vi "MH_AllDllFunctions_AnyThread.vi"   [LabVIEW 2020]
uses:
  mhlib_x86_x64_AnyThread.llb/MH_DllPath_global.vi
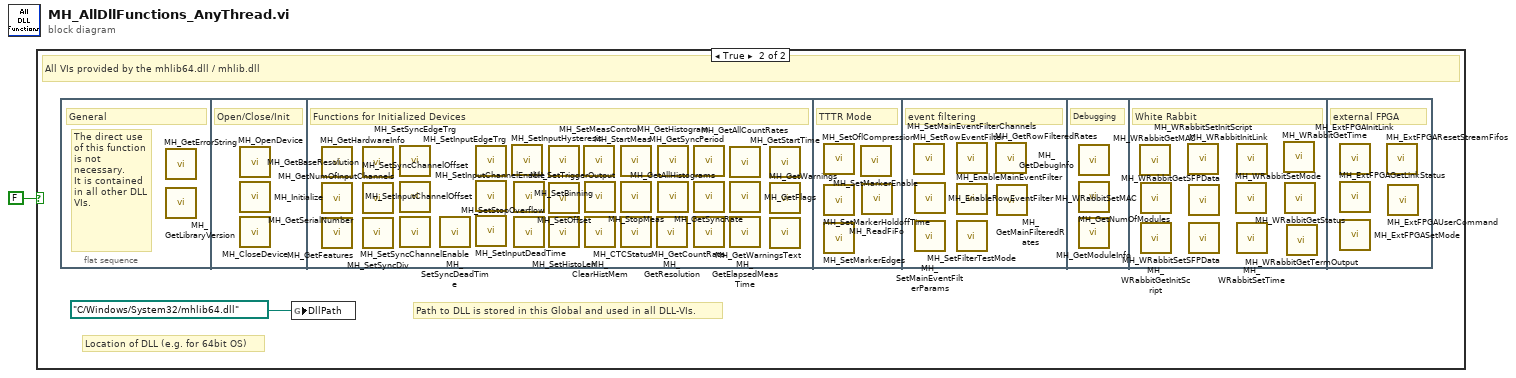
[diagram p0: block diagram]
diagram:
  n1 = case shown="True" FALSE {
    frame False {
    }
    frame True {
      # "Location of DLL (e.g. for 64bit OS)"
      # "Path to DLL is stored in this Global and used in all DLL-VIs."
      # "All VIs provided by the mhlib64.dll / mhlib.dll"
      n2 = flat-sequence {
        frame #0 {
          # "The direct use of this function is not necessary.\nIt is contained in all other DLL VIs."
          # "General"
          n3 = call "MH_GetErrorString.vi"() -> ()  [unwired: 9 in, 3 out]
          n4 = call "MH_GetLibraryVersion.vi"() -> ()  [unwired: 9 in, 3 out]
        }
        frame #1 {
          # "Open/Close/Init"
          n5 = call "MH_OpenDevice.vi"() -> ()  [unwired: 9 in, 3 out]
          n6 = call "MH_Initialize.vi"() -> ()  [unwired: 10 in, 2 out]
          n7 = call "MH_CloseDevice.vi"() -> ()  [unwired: 10 in, 2 out]
        }
        frame #2 {
          # "Functions for Initialized Devices"
          n8 = call "MH_GetHardwareInfo.vi"() -> ()  [unwired: 7 in, 5 out]
          n9 = call "MH_GetSerialNumber.vi"() -> ()  [unwired: 9 in, 3 out]
          n10 = call "MH_GetFeatures.vi"() -> ()  [unwired: 9 in, 3 out]
          n11 = call "MH_GetBaseResolution.vi"() -> ()  [unwired: 8 in, 4 out]
          n12 = call "MH_GetNumOfInputChannels.vi"() -> ()  [unwired: 9 in, 3 out]
          n13 = call "MH_SetSyncDiv.vi"() -> ()  [unwired: 10 in, 2 out]
          n14 = call "MH_SetSyncEdgeTrg.vi"() -> ()  [unwired: 10 in, 2 out]
          n15 = call "MH_SetSyncChannelOffset.vi"() -> ()  [unwired: 10 in, 2 out]
          n16 = call "MH_SetSyncChannelEnable.vi"() -> ()  [unwired: 10 in, 2 out]
          n17 = call "MH_SetSyncDeadTime.vi"() -> ()  [unwired: 10 in, 2 out]
          n18 = call "MH_SetInputEdgeTrg.vi"() -> ()  [unwired: 10 in, 2 out]
          n19 = call "MH_SetInputChannelOffset.vi"() -> ()  [unwired: 10 in, 2 out]
          n20 = call "MH_SetInputDeadTime.vi"() -> ()  [unwired: 10 in, 2 out]
          n21 = call "MH_SetInputHysteresis.vi"() -> ()  [unwired: 10 in, 2 out]
          n22 = call "MH_SetInputChannelEnable.vi"() -> ()  [unwired: 10 in, 2 out]
          n23 = call "MH_SetStopOverflow.vi"() -> ()  [unwired: 10 in, 2 out]
          n24 = call "MH_SetBinning.vi"() -> ()  [unwired: 10 in, 2 out]
          n25 = call "MH_SetOffset.vi"() -> ()  [unwired: 10 in, 2 out]
          n26 = call "MH_SetHistoLen.vi"() -> ()  [unwired: 9 in, 3 out]
          n27 = call "MH_SetMeasControl.vi"() -> ()  [unwired: 10 in, 2 out]
          n28 = call "MH_SetTriggerOutput.vi"() -> ()  [unwired: 10 in, 2 out]
          n29 = call "MH_ClearHistMem.vi"() -> ()  [unwired: 10 in, 2 out]
          n30 = call "MH_StartMeas.vi"() -> ()  [unwired: 10 in, 2 out]
          n31 = call "MH_StopMeas.vi"() -> ()  [unwired: 10 in, 2 out]
          n32 = call "MH_CTCStatus.vi"() -> ()  [unwired: 9 in, 3 out]
          n33 = call "MH_GetResolution.vi"() -> ()  [unwired: 9 in, 3 out]
          n34 = call "MH_GetHistogram.vi"() -> ()  [unwired: 9 in, 3 out]
          n35 = call "MH_GetAllHistograms.vi"() -> ()  [unwired: 9 in, 3 out]
          n36 = call "MH_GetSyncPeriod.vi"() -> ()  [unwired: 9 in, 3 out]
          n37 = call "MH_GetSyncRate.vi"() -> ()  [unwired: 9 in, 3 out]
          n38 = call "MH_GetCountRate.vi"() -> ()  [unwired: 9 in, 3 out]
          n39 = call "MH_GetAllCountRates.vi"() -> ()  [unwired: 8 in, 4 out]
          n40 = call "MH_GetFlags.vi"() -> ()  [unwired: 9 in, 3 out]
          n41 = call "MH_GetElapsedMeasTime.vi"() -> ()  [unwired: 9 in, 3 out]
          n42 = call "MH_GetStartTime.vi"() -> ()  [unwired: 7 in, 5 out]
          n43 = call "MH_GetWarnings.vi"() -> ()  [unwired: 9 in, 3 out]
          n44 = call "MH_GetWarningsText.vi"() -> ()  [unwired: 9 in, 3 out]
        }
        frame #3 {
          # "TTTR Mode"
          n45 = call "MH_SetOflCompression.vi"() -> ()  [unwired: 10 in, 2 out]
          n46 = call "MH_SetMarkerHoldoffTime.vi"() -> ()  [unwired: 10 in, 2 out]
          n47 = call "MH_SetMarkerEdges.vi"() -> ()  [unwired: 10 in, 2 out]
          n48 = call "MH_SetMarkerEnable.vi"() -> ()  [unwired: 10 in, 2 out]
          n49 = call "MH_ReadFiFo.vi"() -> ()  [unwired: 8 in, 4 out]
        }
        frame #4 {
          # "event filtering"
          n50 = call "MH_SetRowEventFilter.vi"() -> ()  [unwired: 10 in, 2 out]
          n51 = call "MH_EnableRowEventFilter.vi"() -> ()  [unwired: 10 in, 2 out]
          n52 = call "MH_SetMainEventFilterParams.vi"() -> ()  [unwired: 10 in, 2 out]
          n53 = call "MH_SetMainEventFilterChannels.vi"() -> ()  [unwired: 10 in, 2 out]
          n54 = call "MH_EnableMainEventFilter.vi"() -> ()  [unwired: 10 in, 2 out]
          n55 = call "MH_SetFilterTestMode.vi"() -> ()  [unwired: 10 in, 2 out]
          n56 = call "MH_GetRowFilteredRates.vi"() -> ()  [unwired: 8 in, 4 out]
          n57 = call "MH_GetMainFilteredRates.vi"() -> ()  [unwired: 8 in, 4 out]
        }
        frame #5 {
          # "Debugging"
          n58 = call "MH_GetDebugInfo.vi"() -> ()  [unwired: 9 in, 3 out]
          n59 = call "MH_GetNumOfModules.vi"() -> ()  [unwired: 9 in, 3 out]
          n60 = call "MH_GetModuleInfo.vi"() -> ()  [unwired: 8 in, 4 out]
        }
        frame #6 {
          # "White Rabbit"
          n61 = call "MH_WRabbitGetMAC.vi"() -> ()  [unwired: 9 in, 3 out]
          n62 = call "MH_WRabbitSetMAC.vi"() -> ()  [unwired: 10 in, 2 out]
          n63 = call "MH_WRabbitGetInitScript.vi"() -> ()  [unwired: 9 in, 3 out]
          n64 = call "MH_WRabbitSetInitScript.vi"() -> ()  [unwired: 10 in, 2 out]
          n65 = call "MH_WRabbitGetSFPData.vi"() -> ()  [unwired: 6 in, 6 out]
          n66 = call "MH_WRabbitSetSFPData.vi"() -> ()  [unwired: 10 in, 2 out]
          n67 = call "MH_WRabbitSetMode.vi"() -> ()  [unwired: 10 in, 2 out]
          n68 = call "MH_WRabbitInitLink.vi"() -> ()  [unwired: 10 in, 2 out]
          n69 = call "MH_WRabbitSetTime.vi"() -> ()  [unwired: 10 in, 2 out]
          n70 = call "MH_WRabbitGetTime.vi"() -> ()  [unwired: 8 in, 4 out]
          n71 = call "MH_WRabbitGetStatus.vi"() -> ()  [unwired: 9 in, 3 out]
          n72 = call "MH_WRabbitGetTermOutput.vi"() -> ()  [unwired: 8 in, 4 out]
        }
        frame #7 {
          # "external FPGA"
          n73 = call "MH_ExtFPGAInitLink.vi"() -> ()  [unwired: 10 in, 2 out]
          n74 = call "MH_ExtFPGAGetLinkStatus.vi"() -> ()  [unwired: 9 in, 3 out]
          n75 = call "MH_ExtFPGASetMode.vi"() -> ()  [unwired: 10 in, 2 out]
          n76 = call "MH_ExtFPGAResetStreamFifos.vi"() -> ()  [unwired: 10 in, 2 out]
          n77 = call "MH_ExtFPGAUserCommand.vi"() -> ()  [unwired: 9 in, 3 out]
        }
      }
      n78 = global write "MH_DllPath_global.vi" "DllPath"(path "C:/Windows/System32/mhlib64.dll" ("DllPath")) -> ()
    }
  }
